vi "otworzI2C.vi"(7 "I2C Channel":u8, 8 "Error In":errorcluster, 10 "I2C Slave Address (0x1D)":u8=29 format="%.0x", 11 "LINX Ref":T1) -> (0 "Error Out":errorcluster, 3 "LINX Resource":T1)   [LabVIEW 2014]
doc: "Open the I2C master and initialize the MMA8452 accelerometer.\n\nIf the LINX device has more than one I2C master the logical first I2C master is channel 0, the next is channel 1, etc."
uses:
  <vilib>/MakerHub/LINX/LMH-LINX.lvlib
  <vilib>/MakerHub/LINX/Private/Type Defs/Peripherals/I2C/EOF.ctl
  czytajI2CVIs/usrednijVIs/AkcjaUsredniania.ctl
  <vilib>/MakerHub/LINX/Private/Type Defs/Platform.ctl
  <vilib>/MakerHub/LINX/Private/Type Defs/Interface.ctl
  <vilib>/MakerHub/LINX/Private/Device/Type Defs/TCP Config.ctl
  <vilib>/MakerHub/LINX/Private/Device/Device.lvlib
  <vilib>/MakerHub/LINX/Private/Device/Type Defs/Channels.ctl
  <vilib>/MakerHub/LINX/Private/Device/Type Defs/LINX Device Config.ctl
  <vilib>/MakerHub/LINX/Private/Type Defs/LINX Ref.ctl
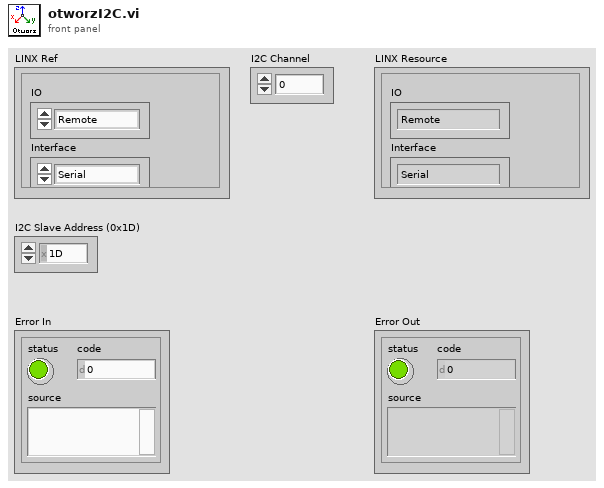
[diagram p1: front panel]
types:
  T1 = typedef "LMH-LINX.lvlib/LINX Ref.ctl" = cluster{"IO":T2, "Interface":T3, "LINX Device Config":T4}
  T2 = typedef "LMH-LINX.lvlib/Platform.ctl" = enum16{"Remote", "Local"}
  T3 = typedef "LMH-LINX.lvlib/Interface.ctl" = enum16{"Serial", "TCP"}
  T4 = typedef "LMH-LINX.lvlib/Device.lvlib/LINX Device Config.ctl" = cluster{"Interface":T3, "COM Port":refnum<visa-resource-name>, "TCP Configuration":T5, "Device Family":u8, "Device ID":u8, "Device Name":string, "TCP Ref":refnum<k5>, "Channels":T6}
  T5 = typedef "LMH-LINX.lvlib/Device.lvlib/TCP Config.ctl" = cluster{"IP Address":string, "Port":u16}
  T6 = typedef "LMH-LINX.lvlib/Channels.ctl" = cluster{"DI":u8[], "DO":u8[], "AI":u8[], "AO":u8[], "PWM":u8[], "QE":u8[], "UART":u8[], "I2C 2":u8[], "SPI":u8[], "CAN":u8[], "Servo":u8[], "AI Ref (V)":dbl, "AI Resolution (Bits)":u8, "AO Ref (V)":dbl, "AO Resolution (Bits)":u8}
  T7 = typedef "LMH-LINX.lvlib/EOF.ctl" = enum8{"Stop", "Restart", "Restart No Stop", "No Stop"}
  T8 = typedef "AkcjaUsredniania.ctl" = enum16{"Init", "DodajWartość", "WypełnijKolejkę", "Czyść"}
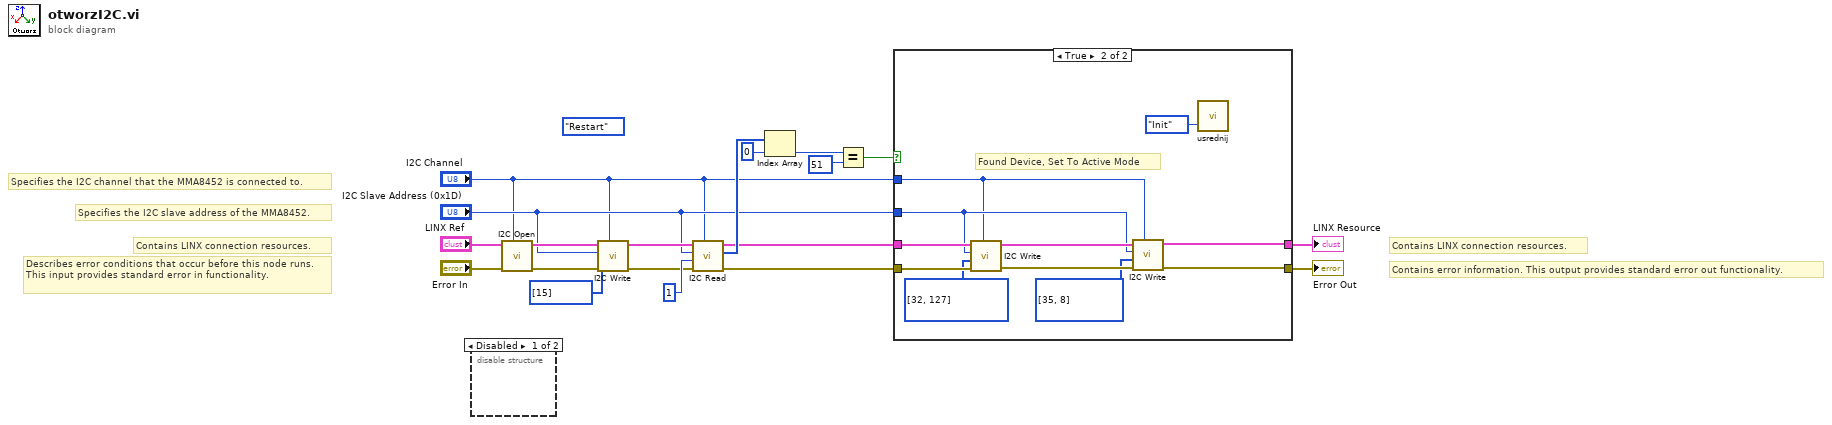
[diagram p0: block diagram]
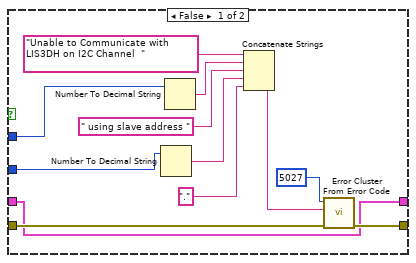
[diagram p3: hidden frame]
diagram:
  (unwired) EOF."Restart" ("EOF")
  # "Contains LINX connection resources."
  # "Contains error information. This output provides standard error out functionality."
  # "Specifies the I2C slave address of the MMA8452."
  # "Specifies the I2C channel that the MMA8452 is connected to."
  # "Contains LINX connection resources."
  # "Describes error conditions that occur before this node runs. This input provides standard error in functionality."
  n1 = disable-structure shown="Disabled" {
    frame Disabled {
    }
    frame Enabled {
    }
  }
  n2 = call <vilib>:"I2C Open.vi"("I2C Channel (0)"="I2C Channel", "Error In"="Error In", "LINX Resource"="LINX Ref") -> ("Error Out"=w5:errorcluster, "LINX Resource"=w7:T1)  [unwired: 7 in]
  n3 = call <vilib>:"I2C Write.vi"("I2C Channel"="I2C Channel", "Error In"=w5, "Data"=u8[] [15], "I2C Slave Address (0)"="I2C Slave Address (0x1D)", "LINX Resource"=w7) -> ("Error Out"=w4:errorcluster, "LINX Resource"=w6:T1)  [unwired: 5 in]
  n4 = call <vilib>:"I2C Read.vi"("I2C Channel"="I2C Channel", "Error In"=w4, "Bytes To Read"=u8 1, "I2C Slave Address (0)"="I2C Slave Address (0x1D)", "LINX Resource"=w6) -> ("Error Out"=w11:errorcluster, "Data"=w16:u8[], "LINX Resource"=w10:T1)  [unwired: 4 in]
  n5 = Index Array(array=w16, index=0) -> (element=w18:u8)
  n6 = Equal?(x=w18, y=u8 51) -> (x = y?=w12:bool)
  n7 = case shown="True" w12 {
    tunnel: w11 -> [w25 w41]
    tunnel: w10 -> [w20 w42]
    tunnel: [w23 w36] -> w9
    tunnel: "I2C Channel" -> [w22 w34]
    tunnel: "I2C Slave Address (0x1D)" -> [w21 w35]
    tunnel: [w20 w37] -> w8
    frame False {
      n8 = Number To Decimal String(number=w21) -> (decimal integer string=w30:string)  [unwired: 1 in]
      n9 = Number To Decimal String(number=w22) -> (decimal integer string=w28:string)  [unwired: 1 in]
      n10 = Concatenate Strings("Unable to Communicate with LIS3DH on I2C Channel  " ("error message (\"\")"), w28, " using slave address " ("string"), w30, "." ("string")) -> (w24:string)
      n11 = call <vilib>:"Error Cluster From Error Code.vi"("error in (no error)"=w25, "error message (\"\")"=w24, "error code (0)"=5027) -> ("error out"=w23:errorcluster)  [unwired: 6 in]
    }
    frame True {
      # "Found Device, Set To Active Mode"
      n12 = call <vilib>:"I2C Write.vi"("I2C Channel"=w34, "Error In"=w41, "Data"=u8[] [32, 127], "I2C Slave Address (0)"=w35, "LINX Resource"=w42) -> ("Error Out"=w38:errorcluster, "LINX Resource"=w39:T1)  [unwired: 5 in]
      n13 = call <vilib>:"I2C Write.vi"("I2C Channel"=w34, "Error In"=w38, "Data"=u8[] [35, 8], "I2C Slave Address (0)"=w35, "LINX Resource"=w39) -> ("Error Out"=w36:errorcluster, "LINX Resource"=w37:T1)  [unwired: 5 in]
      n14 = call "usrednij.vi"("AkcjaUsredniania"=AkcjaUsredniania."Init") -> ()  [unwired: 1 in, 2 out]
    }
  }
  "LINX Resource" <- w8
  "Error Out" <- w9
